vi "Disable Motor.vi"(8 "Error In":errorcluster, 10 "Enable Channel":u8=11, 11 "Serial Port":refnum<visa-resource-name>="COM6") -> (0 "error out":errorcluster)   [LabVIEW 2016]
uses:
  <vilib>/MakerHub/LINX/Public/Peripherals/Digital/Digital Write 1 Chan.vi
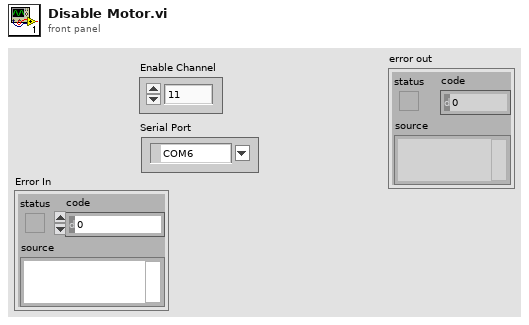
[diagram p1: front panel]
types:
  T1 = typedef "LMH-LINX.lvlib/LINX Ref.ctl" = cluster{"Platform":T2, "Interface":T3, "LINX Device Config":T4}
  T2 = typedef "LMH-LINX.lvlib/Platform.ctl" = enum16{"LINX", "myRIO"}
  T3 = typedef "LMH-LINX.lvlib/Interface.ctl" = enum16{"Serial", "TCP"}
  T4 = typedef "LMH-LINX.lvlib/Device.lvlib/LINX Device Config.ctl" = cluster{"Interface":T3, "COM Port":refnum<visa-resource-name>, "TCP Configuration":T5, "Device Family":u8, "Device ID":u8, "Device Name":string, "TCP Ref":refnum<k5>, "Channels":T6}
  T5 = typedef "LMH-LINX.lvlib/Device.lvlib/TCP Config.ctl" = cluster{"IP Address":string, "Port":u16}
  T6 = typedef "LMH-LINX.lvlib/Channels.ctl" = cluster{"DI":u8[], "DO":u8[], "AI":u8[], "AO":u8[], "PWM":u8[], "QE":u8[], "UART":u8[], "I2C 2":u8[], "SPI":u8[], "CAN":u8[], "Servo":u8[], "AI Ref (V)":dbl, "AO Ref (V)":dbl, "AO Resolution (Bits)":u8}
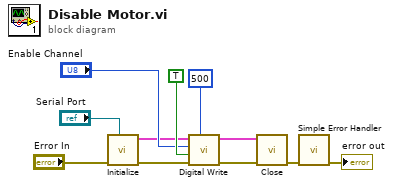
[diagram p0: block diagram]
diagram:
  n1 = call <vilib>:"Initialize.vi"("Serial Port"="Serial Port", "Error In"="Error In") -> ("Error Out"=w5:errorcluster, "LINX Ref"=w6:T1)  [unwired: 7 in, 1 out]
  n2 = call-poly <vilib>:"Digital Write.vi"("Timeout (100 ms)"=500, "Error In"=w5, "Output Value"=TRUE ("LED Value"), "DO Channel"="Enable Channel", "LINX Resource"=w6) -> ("Error Out"=w3:errorcluster, "LINX Resource"=w4:T1)  [unwired: 5 in]
  n3 = call <vilib>:"Close.vi"("Error In"=w3, "LINX Resource"=w4) -> ("Error Out"=w8:errorcluster)  [unwired: 8 in, 1 out]
  n4 = call <vilib>:"Simple Error Handler.vi"("error in (no error)"=w8) -> ("error out"=→"error out":errorcluster)  [unwired: 4 in, 4 out]
